vi "DisconnectAll.vi"(8 "error in (no error)":errorcluster, 10 "gRPCid":T2, 11 "ctet_mux in":T1) -> (0 "error out":errorcluster, 3 "ctet_mux out":T1)   [LabVIEW 2019, in "ctet_mux_User Library.lvlib"]
uses:
  ctet_mux_User Library.lvlib
  Servers/ctet_mux/gRPC lvSupport/Server API/typeDefs/grpcId.ctl
  Types/ctet_mux.ctl
  Servers/ctet_mux/ctet_mux Class/RPC Messages/measurementservice_MUXDisconnectAllResponse/measurementservice_MUXDisconnectAllResponse_Data.ctl
  Servers/ctet_mux/ctet_mux Class/RPC Messages/measurementservice_ErrorOut/measurementservice_ErrorOut_Data.ctl
  Servers/ctet_mux/ctet_mux Class/ctet_mux.lvclass
  Servers/ctet_mux/gRPC lvSupport/gprc-lvsupport.lvlib
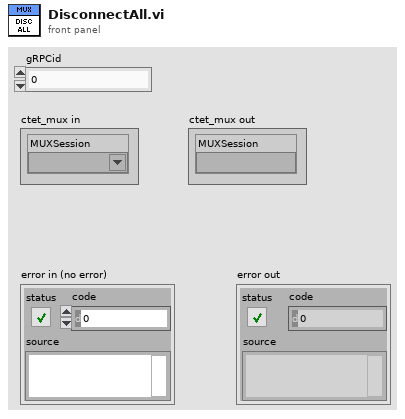
[diagram p1: front panel]
types:
  T1 = typedef "ctet_mux_User Library.lvlib/ctet_mux.ctl" = cluster{"MUXSession":refnum<k15>}
  T2 = typedef "ctet_mux.lvlib/gprc-lvsupport.lvlib/grpcId.ctl" = u64
  T3 = typedef "ctet_mux.lvlib/ctet_mux.lvclass/measurementservice_ErrorOut_Data.ctl" = cluster{"errCode":i64, "errMessage":string}
  T4 = typedef "ctet_mux.lvlib/ctet_mux.lvclass/measurementservice_MUXDisconnectAllResponse_Data.ctl" = cluster{"error":T3}
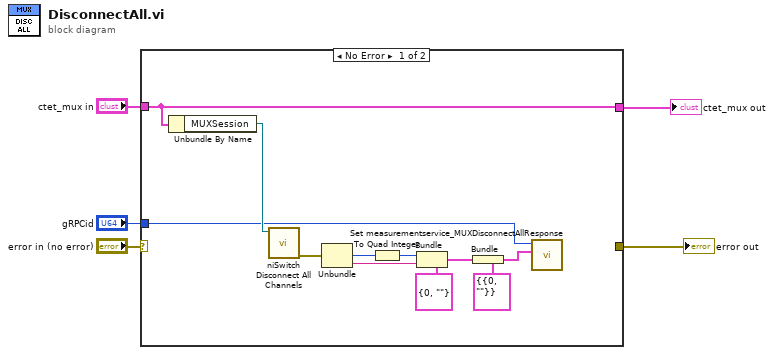
[diagram p0: block diagram]
diagram:
  n1 = case shown="No Error" "error in (no error)" {
    selector: "error in (no error)" -> [_ w18]
    tunnel: [_ w18] -> w5
    tunnel: "gRPCid" -> [w10 _]
    tunnel: "ctet_mux in" -> [w11 w17]
    tunnel: [w11 w17] -> w1
    frame No Error {
      n2 = Unbundle By Name(w11) -> ("MUXSession"=w12:refnum<k15>)
      n3 = call <instrlib>:"niSwitch Disconnect All Channels.vi"("instrument handle"=w12) -> ("error out"=w16:errorcluster)  [unwired: 9 in, 1 out]
      n4 = Unbundle(w16) -> ("code"=w14:i32, "source"=w15:string)  [unwired: 1 out]
      n5 = To Quad Integer(1:w14) -> (0:w13:i64)
      n6 = Bundle(cluster=T3 {"errCode"=0, "errMessage"=""} ("error"), "errCode"=w13, "errMessage"=w15) -> (w6:T3)
      n7 = Bundle(cluster=T4 {"error"={"errCode"=0, "errMessage"=""}} ("Message Data"), "error"=w6) -> (w8:T4)
      n8 = call "Set measurementservice_MUXDisconnectAllResponse.vi"("Message Data"=w8, "gRPCid"=w10) -> ()  [unwired: 9 in, 1 out]
    }
    frame Error {
    }
  }
  "error out" <- w5
  "ctet_mux out" <- w1
